vi "WPC Stats Main.vi"() -> ()   [LabVIEW 2021]
uses:
  SubVIs/WPC Player and Financial Stats.ctl
panel:
  out "residual":dbl format="%03.2f"
  out "Sorted by profit":cluster{"Player Name":string, "Profit":dbl}[](array[cluster]) {"Profit" format="%#.2g"}
  out "Stats since last update":T1[](array[typedef]) {"Date Updated" format="%<%m/%d/%Y>T"}
  in  "Back up data file?":bool=TRUE
  in  "file path (use dialog)":path=path "C:/Users/manma/Google Drive/WPC Stat Scrape/Data/WPC Stats.bin"
  out "File updated?":bool
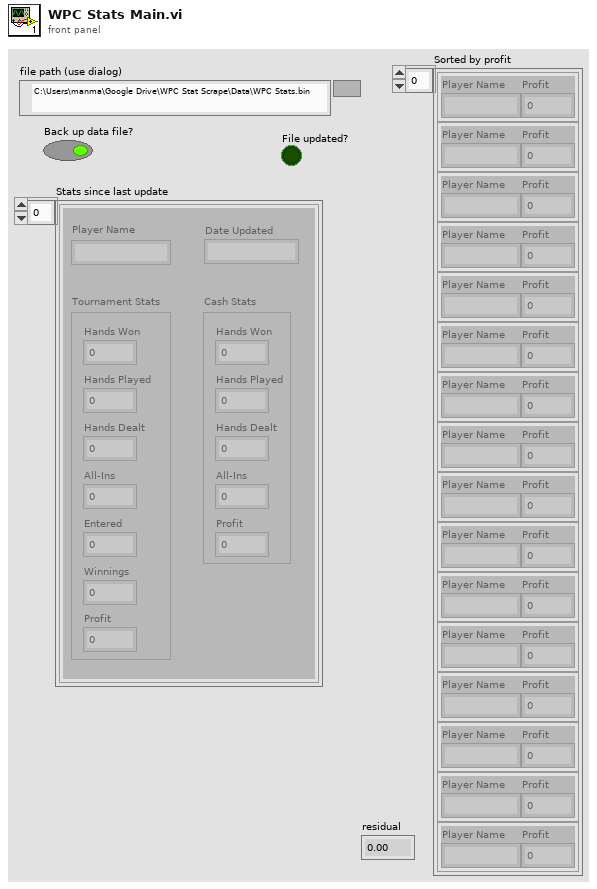
[diagram p1: front panel]
types:
  T1 = typedef "WPC Player and Financial Stats.ctl" = cluster{"Player Name":string, "Date Updated":timestamp, "Tournament Stats":cluster{"Hands Won":i32, "Hands Played":i32, "Hands Dealt":i32, "All-Ins":i32, "Entered":i32, "Winnings":dbl, "Profit":dbl}, "Cash Stats":cluster{"Hands Won":i32, "Hands Played":i32, "Hands Dealt":i32, "All-Ins":i32, "Profit":dbl}}
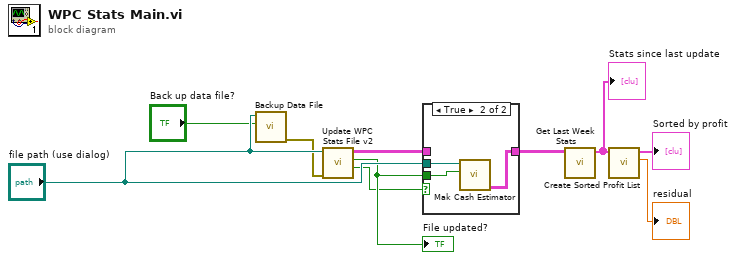
[diagram p0: block diagram]
diagram:
  n1 = call "Backup Data File.vi"("Back up data file?"="Back up data file?", "file path (use dialog)"="file path (use dialog)") -> ("error out"=w2:errorcluster)  [unwired: 9 in]
  n2 = call "Update WPC Stats File v2.vi"("error in (no error)"=w2, "file path (use dialog)"="file path (use dialog)") -> ("redacted?"=w7:bool, "File Updated?"=w8:bool, "Full WPC Stats"=w6:T1[][])  [unwired: 6 in, 1 out]
  "File updated?" <- w8
  n3 = case shown="True" w7 {
    tunnel: "file path (use dialog)" -> [_ w14]
    tunnel: [w11 w13] -> w9
    tunnel: w8 -> [_ w12]
    tunnel: w6 -> [w11 _]
    frame False {
    }
    frame True {
      n4 = call "Mak Cash Estimator.vi"("Update Stats File?"=w12, "file path (use dialog)"=w14) -> ("Full WPC Stats"=w13:T1[][])  [unwired: 6 in, 3 out]
    }
  }
  n5 = call "Get Last Week Stats.vi"("WPC Stats"=w9) -> ("Last Week's Stats"=w5:T1[])  [unwired: 10 in]
  "Stats since last update" <- w5
  n6 = call "Create Sorted Profit List.vi"("Stats since last update"=w5) -> ("residual"=→"residual":dbl, "Sorted by profit"=→"Sorted by profit":cluster{"Player Name":string, "Profit":dbl}[])  [unwired: 9 in]
